vi "SlobalState.vi"() -> ()   [LabVIEW 2016]
uses:
  TestControl.ctl
panel:
  in  "Cluster":T1
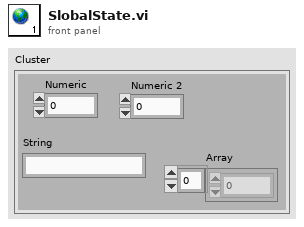
[diagram p1: front panel]
types:
  T1 = typedef "TestControl.ctl" = cluster{"Array":dbl[], "String":string, "Numeric":dbl, "Numeric 2":dbl}
diagram:
